vi "_emi_GFV Loop Linking.vi"(0 "Loop Index/Numb":u16, 1 "Action(Get Index)":T1=enum."Get index", 7 "Linked indexes in":u16[](array[numeric]), 11 "error in (no error)":errorcluster) -> (4 "Index out":u16, 8 "Linked indexes out":u16[](array[numeric]), 10 "Size":i32, 15 "error out":errorcluster)   [LabVIEW 2011]
uses:
  _emi_Loop control int action.ctl
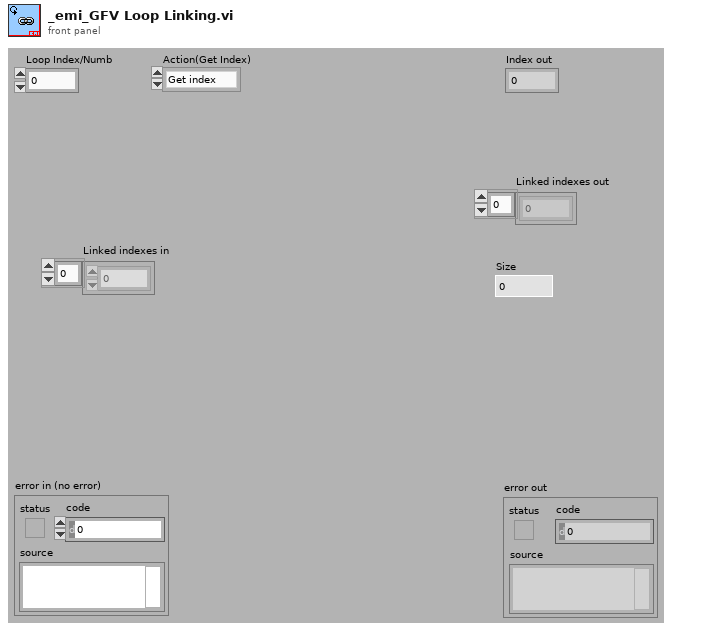
[diagram p1: front panel]
types:
  T1 = typedef "_emi_Loop control int action.ctl" = enum16{"Init index", "Get index", "Set index", "Get Size"}
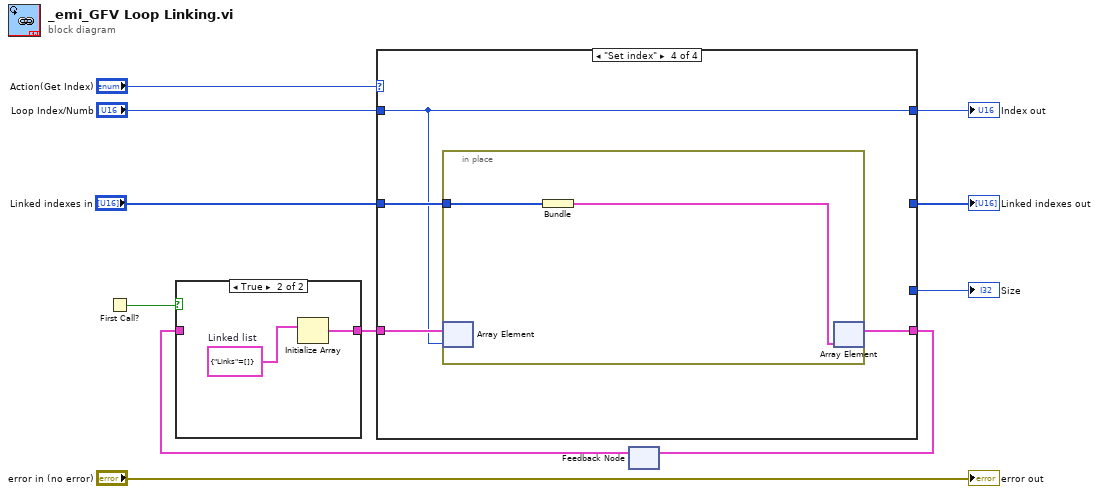
[diagram p0: block diagram]
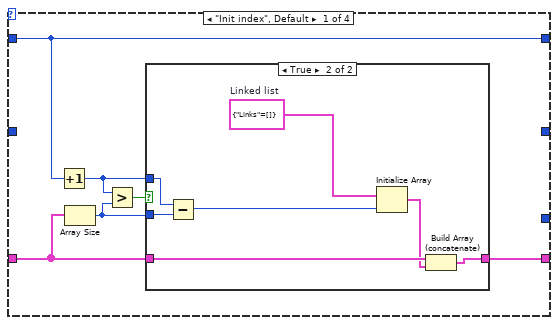
[diagram p2: hidden frame]
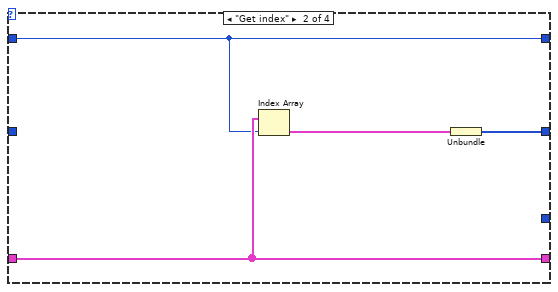
[diagram p4: hidden frame]
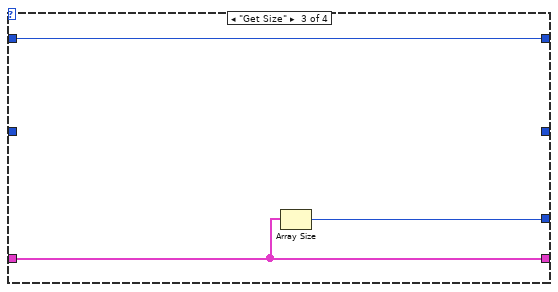
[diagram p5: hidden frame]
diagram:
  n1 = First Call?() -> (First Call?: T/F=w11:bool)
  n2 = feedback #1() -> (w5:cluster{"Links":u16[]}[])  [unwired: 1 in]
  n3 = case shown="True" w11 {
    tunnel: [w12 w13] -> w6
    tunnel: w5 -> [w12 _]
    frame False {
    }
    frame True {
      w14 = cluster{"Links":u16[]} {"Links"=[]}  # Linked list
      n4 = Initialize Array(w14) -> (w13:cluster{"Links":u16[]}[])  [unwired: 1 in]
    }
  }
  n5 = case shown="\"Set index\"" "Action(Get Index)" {
    tunnel: [w20 w31 w35 w36] -> w10
    tunnel: "Loop Index/Numb" -> [w20 w31 w35 w36]
    tunnel: [w16 w32 w34 w38] -> w7
    tunnel: w6 -> [w15 w32 w34 w39]
    tunnel: [_ w29 _ _] -> w1
    tunnel: "Linked indexes in" -> [_ _ _ w37]
    tunnel: [_ _ w33 _] -> w3
    frame "Init index", Default {
      n6 = Increment(x=w20) -> (x+1=w17:u16)
      n7 = Array Size(array=w15) -> (size(s)=w18:i32)
      n8 = Greater?(x=w17, y=w18) -> (0:w19:bool)
      n9 = case shown="True" w19 {
        tunnel: w18 -> [_ w27]
        tunnel: w17 -> [_ w28]
        tunnel: [w21 w23] -> w16
        tunnel: w15 -> [w21 w25]
        frame False {
        }
        frame True {
          w22 = cluster{"Links":u16[]} {"Links"=[]}  # Linked list
          n10 = Subtract(x=w28, y=w27) -> (x-y=w26:i32)
          n11 = Initialize Array(w22, w26) -> (w24:cluster{"Links":u16[]}[])
          n12 = Build Array (concatenate)(w25, w24) -> (w23:cluster{"Links":u16[]}[])
        }
      }
    }
    frame "Get index" {
      n13 = Index Array(array=w32, index=w31) -> (element=w30:cluster{"Links":u16[]})
      n14 = Unbundle(w30) -> ("Links"=w29:u16[])
    }
    frame "Get Size" {
      n15 = Array Size(array=w34) -> (size(s)=w33:i32)
    }
    frame "Set index" {
      n16 = in-place {
        in-place-border: w37 -> [w41]
        n17 = in-place-array #2(w39, w36) -> ()  [unwired: 1 out]
        n18 = Bundle("Linked indexes in"=w41) -> (w40:cluster{"Linked indexes in":u16[]})  [unwired: 1 in]
        n19 = in-place-array #2(w40) -> (w38:cluster{"Links":u16[]}[])  [unwired: 1 out]
      }
    }
  }
  "Index out" <- w10
  "Size" <- w3
  "Linked indexes out" <- w1
  n20 = feedback-in #1(w7) -> ()
  "error out" <- "error in (no error)"
